vi "GetStringValue.vi"(8 "error in (no error)":errorcluster caption="错误输入（无错误）", 10 "strKey":string, 11 "handle":u64) -> (0 "error out":errorcluster caption="错误输出", 2 "function return":i32, 3 "handle out":u64)   [LabVIEW 2011, in "MvCameraControl.lvlib"]
doc: "MV_LV_API int __stdcall GetStringValue( void* handle, const char* strKey, MVCC_STRINGVALUE *pStringValue);"
uses:
  MvCameraControl.lvlib
  MvCameraPatch.dll
panel:
  out "pStringValue":T1
  in  "StringValue":T1
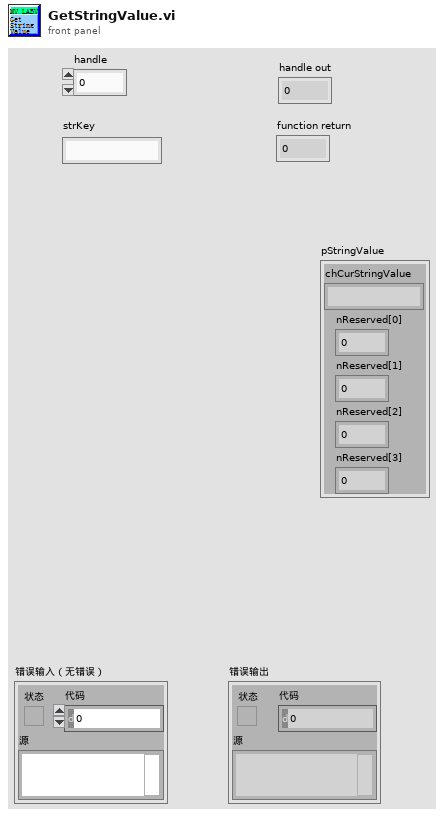
[diagram p1: front panel]
types:
  T1 = cluster{"chCurStringValue":string, "nReserved[0]":u32, "nReserved[1]":u32, "nReserved[2]":u32, "nReserved[3]":u32}
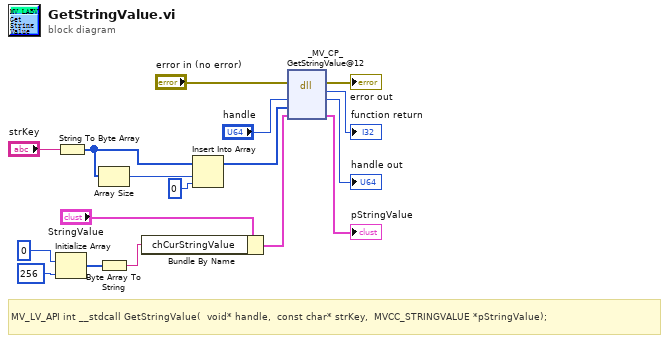
[diagram p0: block diagram]
diagram:
  # "MV_LV_API int __stdcall GetStringValue(  void* handle,  const char* strKey,  MVCC_STRINGVALUE *pStringValue);"
  n1 = Initialize Array(u8 0 ("元素"), 256 ("维数大小")) -> (w6:u8[])
  n2 = String To Byte Array(string="strKey") -> (unsigned byte array=w13:u8[])
  n3 = Array Size(array=w13) -> (size(s)=w12:i32)
  n4 = Byte Array To String(unsigned byte array=w6) -> (string=w7:string)
  n5 = Bundle By Name(cluster="StringValue", "chCurStringValue"=w7) -> (w3:T1)
  n6 = Insert Into Array(array=w13, index=w12, new element=u8 0 ("新元素/子数组")) -> (w9:u8[])
  n7 = dll-call lib="MvCameraPatch.dll" fn="_MV_CP_GetStringValue@12"(error in="error in (no error)", "handle"="handle", "strKey"=w9, "pStringValue"=w3) -> (error out=→"error out":errorcluster, "返回类型"=→"function return":i32, "handle"=→"handle out":u64, "pStringValue"=→"pStringValue":T1)  [unwired: 3 in, 1 out]
